vi "Actor Core.vi"(8 "error in":errorcluster, 11 "Launch IMAQ Display in":refnum<class "Launch File Viewer.lvclass">) -> (0 "error out":errorcluster={"status"=FALSE, "code"=0, "source"="Actor Framework.lvlib:Actor.lvclass:Launch Nested Actor.vi<APPEND>\n\n<b>Complete call chain:</b>\r\n     Actor Framework.lvlib:Actor.lvclass:Launch Nested Actor.vi\r\n     Launch HIJ FileViewer.lvlib:Launch File Viewer.lvclass:Actor Core.vi"}, 3 "Actor out":refnum<class "Actor.lvclass">)   [LabVIEW 2014, in "Launch HIJ FileViewer.lvlib" / "Launch File Viewer.lvclass"]
doc: "(<B>Filename</B>: Actor Framework.lvlib:Actor.lvclass:Actor Core.vi)\n\nReceives messages to the actor, reacts to them, and initiates any error handling that may shut the actor down.\n\nDescendant classes may override this VI to append parallel tasks for the actor to complete while it handles messages. Overrides use the Call Parent Method node."
uses:
  Launch File Viewer.lvclass
  <vilib>/ActorFramework/Actor/Actor.lvclass
  Analyze Actor/Analyze Actor/Analyze Actor.lvclass
  HIJ Vision Display/HIJ Vision Display Messages/New Results Msg/New Results Msg.lvclass
  HIJ Vision File Viewer/HIJ Vision File Viewer/HIJ Vision File Viewer.lvclass
  Results and Overlays/Results q-Factor/Analyze Results q-Factor.lvclass
  Analyze Classes/Analyze Fluence/Analyze Fluence.lvclass
  Results and Overlays/Results Fluence/Analyze Results Fluence.lvclass
  Results and Overlays/Results Base/Analyze Results Base.lvclass/Analyze Results Base.ctl
  HIJ Vision Display/HIJ Vision Display/HIJ Vision Display.lvclass/HIJ Vision Display.ctl
  Analyze Actor/Analyze Actor/Analyze Actor.lvclass/Analyze Actor.ctl
  <vilib>/ActorFramework/Actor/Actor.lvclass/Actor.ctl
  <vilib>/ActorFramework/Message Enqueuer/Message Enqueuer.lvclass/Message Enqueuer.ctl
  HIJ Vision Display/HIJ Vision Display Messages/Write Analyze Actor Msg/Write Analyze Enq Msg.lvclass/Write Analyze Enq Msg.ctl
  Shared Code/Viewable Actor/ViewableActor Messages/Insert Into SubPanel Msg/Insert Into SubPanel Msg.lvclass/Insert Into SubPanel Msg.ctl
  HIJ Vision File Viewer/HIJ Vision File Viewer Messages/Load Image from File Msg/Load Image from File Msg.lvclass/Load Image from File Msg.ctl
  Analyze Parameter/Analyze Parameter Energy/Analyze Parameter Energy.lvclass
  Analyze Parameter/Analyze Parameter Fluence/Analyze Parameter Fluence.lvclass
  Analyze Parameter/Analyze Parameter Energy/Analyze Parameter Energy.lvclass/Analyze Parameter Energy.ctl
  Analyze Actor/Analyze Actor Messages/Set Analyze Parameter Msg/Set Analyze Parameter Msg.lvclass/Set Analyze Parameter Msg.ctl
  Analyze Parameter/Analyze Parameter Energy/Write Energy.vi
  Results and Overlays/Results Base/Write Overlay_.vi
  Results and Overlays/Results Base/Write Overlay colors.vi
  HIJ Vision Display/HIJ Vision Display/Write Save Report_.vi
  HIJ Vision Display/HIJ Vision Display/Write Show ZoomBtn_.vi
  HIJ Vision Display/HIJ Vision Display/Write WorkDir.vi
  Analyze Actor/Analyze Actor/Write Analyze Objects.vi
  Analyze Actor/Analyze Actor/Write Publish Analyze Results Msg.vi
  Analyze Actor/Analyze Actor/Write Destination.vi
  <vilib>/ActorFramework/Message Enqueuer/Init from Existing Queue.vi
  <vilib>/ActorFramework/Message Enqueuer/Enqueue.vi
  <vilib>/ActorFramework/Message Priority Queue/Priority Enqueue.vi
  <vilib>/ActorFramework/Message Enqueuer/Message Enqueuer.lvclass
  HIJ Vision Display/HIJ Vision Display Messages/Write Analyze Actor Msg/Write Analyze Enq Msg.lvclass
  Shared Code/Viewable Actor/ViewableActor Messages/Insert Into SubPanel Msg/Insert Into SubPanel Msg.lvclass
  <vilib>/ActorFramework/Stop Msg/Stop Msg.lvclass
  HIJ Vision File Viewer/HIJ Vision File Viewer Messages/Load Image from File Msg/Load Image from File Msg.lvclass
  Analyze Actor/Analyze Actor Messages/Set Analyze Parameter Msg/Set Analyze Parameter Msg.lvclass
  HIJ Vision Display/HIJ Vision Display Messages/Evaluate with new Params Msg/Evaluate with new Params Msg.lvclass
  Shared Code/Viewable Actor/ViewableActor/ViewableActor.lvclass
panel:
  in  "Load Image Report":bool
  in  "Size of region (px)":i32=10
  in  "Energy":dbl[unit] format="%#_13g"
  in  "Image":path=path "C:/Users/user/Desktop/test/WorkDir"
  in  "Stop Button":bool=TRUE
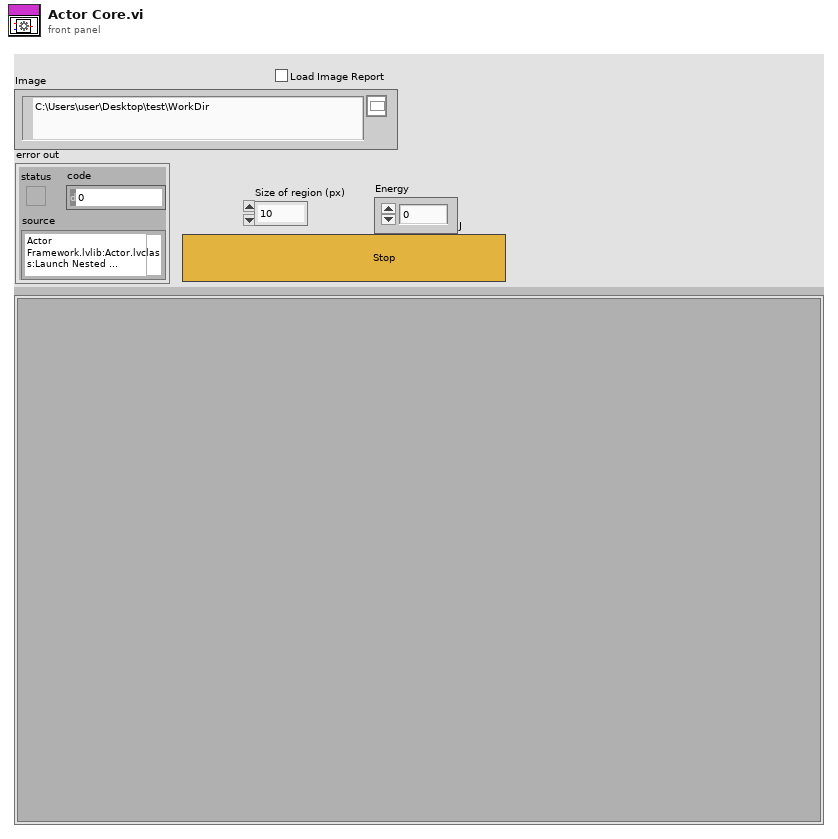
[diagram p1: front panel]
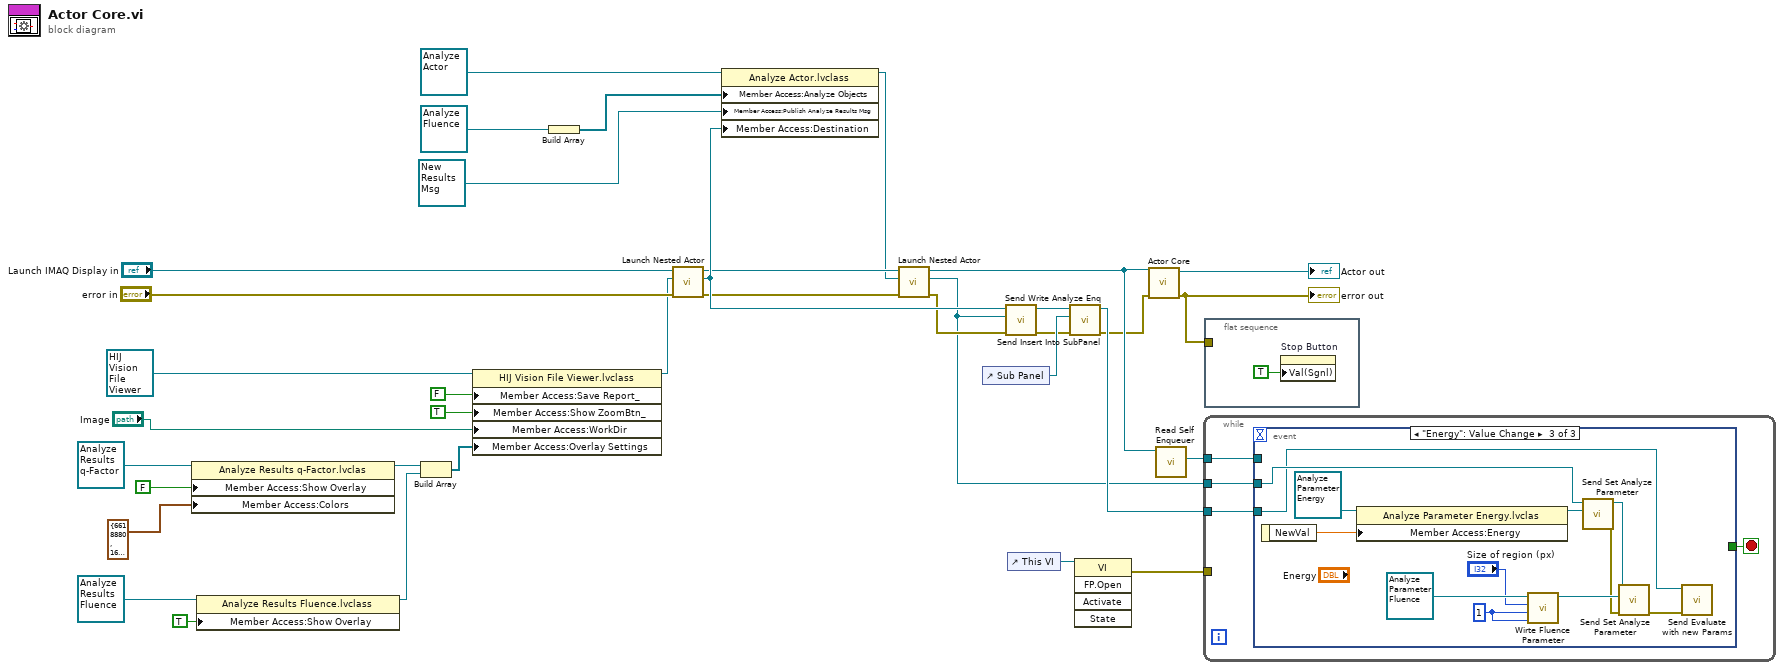
[diagram p0: block diagram]
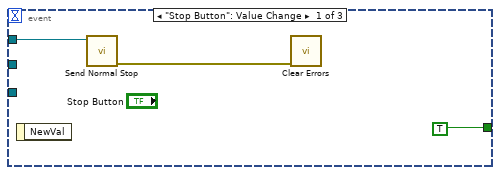
[diagram p2: hidden frame]
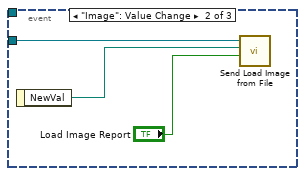
[diagram p3: hidden frame]
diagram:
  n1 = property class="Analyze Results q-Factor.lvclas"(reference=refnum<class "Analyze Results q-Factor.lvclass"> refnum ("Analyze Results q-Factor.lvclass"), "Member Access:Show Overlay"=FALSE ("bOverlay"), "Member Access:Colors"=cluster{"Border":u32, "Text":u32} {"Border"=6618880, "Text"=16448250} ("Colors")) -> (reference out=w9:refnum<class "Analyze Results q-Factor.lvclass">)  [unwired: 1 in, 1 out]
  n2 = property class="Analyze Results Fluence.lvclass"(reference=refnum<class "Analyze Results Fluence.lvclass"> refnum ("Analyze Results Fluence.lvclass"), "Member Access:Show Overlay"=TRUE ("Show Overlay")) -> (reference out=w1:refnum<class "Analyze Results Fluence.lvclass">)  [unwired: 1 in, 1 out]
  n3 = Build Array(w9, w1) -> (w11:refnum<class "Analyze Results Base.lvclass">[])
  n4 = property class="HIJ Vision File Viewer.lvclass"(reference=refnum<class "HIJ Vision File Viewer.lvclass"> refnum ("HIJ Vision File Viewer.lvlib:HIJ Vision File Viewer.lvclass"), "Member Access:Save Report_"=FALSE ("Save Report_"), "Member Access:Show ZoomBtn_"=TRUE ("Show ZoomBtn_"), "Member Access:WorkDir"="Image", "Member Access:Overlay Settings"=w11) -> (reference out=w24:refnum<class "HIJ Vision File Viewer.lvclass">)  [unwired: 1 in, 1 out]
  n5 = Build Array(refnum<class "Analyze Fluence.lvclass"> refnum ("Analyze.lvlib:Analyze Fluence.lvclass")) -> (w20:refnum<class "Analyze Fluence.lvclass">[])
  n6 = call <vilib>:"Launch Nested Actor.vi"("error in (no error)"="error in", "Nested Actor"=w24, "Caller Actor in"="Launch IMAQ Display in") -> ("error out"=w25:errorcluster, "Nested Actor's Enqueuer"=w36:refnum<class "Message Enqueuer.lvclass">, "Caller Actor out"=w18:refnum<class "Launch File Viewer.lvclass">)  [unwired: 6 in]
  n7 = property class="Analyze Actor.lvclass"(reference=refnum<class "Analyze Actor.lvclass"> refnum ("Analyze Actor.lvlib:Analyze Actor.lvclass"), "Member Access:Analyze Objects"=w20, "Member Access:Publish Analyze Results Msg"=refnum<class "New Results Msg.lvclass"> refnum ("HIJ Vision Display.lvlib:New Results Msg.lvclass"), "Member Access:Destination"=w36) -> (reference out=w16:refnum<class "Analyze Actor.lvclass">)  [unwired: 1 in, 1 out]
  n8 = call <vilib>:"Launch Nested Actor.vi"("error in (no error)"=w25, "Nested Actor"=w16, "Caller Actor in"=w18) -> ("error out"=w14:errorcluster, "Nested Actor's Enqueuer"=w5:refnum<class "Message Enqueuer.lvclass">, "Caller Actor out"=w17:refnum<class "Launch File Viewer.lvclass">)  [unwired: 6 in]
  n9 = control-ref of="Sub Panel"() -> (w34:refnum<vi>)
  n10 = call "Send Write Analyze Enq.vi"("error in (no error)"=w14, "Actor Framework:Message Enqueuer"=w5, "Message Enqueuer"=w36) -> ("error out"=w13:errorcluster, "Message Enqueuer out"=w15:refnum<class "Message Enqueuer.lvclass">)  [unwired: 7 in]
  n11 = control-ref of="This VI"() -> (w28:refnum<vi>)
  n12 = call "Send Insert Into SubPanel.vi"("error in (no error)"=w13, "SubPanel Ref"=w34, "Message Enqueuer"=w15) -> ("error out"=w12:errorcluster, "Message Enqueuer out"=w23:refnum<class "Message Enqueuer.lvclass">)  [unwired: 7 in]
  n13 = invoke class="VI" method="FP.Open"(reference=w28) -> (error out=w22:errorcluster)  [unwired: 4 in, 4 out]
  n14 = call-parent "Actor Core.vi"("error in"=w12, "Actor in"=w17) -> ("error out"=w33:errorcluster, "Actor out"=→"Actor out":refnum<class "Actor.lvclass">)  [unwired: 8 in]
  "error out" <- w33
  n15 = call <vilib>:"Read Self Enqueuer.vi"("Actor"=w17) -> ("Self Enqueuer"=w32:refnum<class "Message Enqueuer.lvclass">)  [unwired: 10 in]
  n16 = while {
    tunnel: w32 -> [w39]
    tunnel: w23 -> [w38]
    tunnel: w22 -> [_]
    tunnel: w5 -> [w37]
    stop <- w40 stop-if-true
    n17 = event shown="[2] \"Energy\": Value Change" {
      selector: _ -> [_ _ _]
      dyn-events: _ -> [_ _ _]
      timeout: _ -> [_ _ _]
      tunnel: [TRUE _ _] -> w40
      tunnel: w39 -> [w42 _ _]
      tunnel: w38 -> [_ w46 w55]
      tunnel: w37 -> [_ _ w56]
      event "Stop Button": Value Change {
        n18 = event-data() -> ()  [unwired: 1 in, 1 out]
        n19 = call <vilib>:"Send Normal Stop.vi"("Message Enqueuer"=w42) -> ("error out"=w41:errorcluster)  [unwired: 10 in]
        n20 = call <vilib>:"Clear Errors.vi"("error in (no error)"=w41) -> ()  [unwired: 5 in, 2 out]
      }
      event "Image": Value Change {
        n21 = event-data() -> ("NewVal"=w45:path)  [unwired: 1 in]
        n22 = call "Send Load Image from File.vi"("Load Report"="Load Image Report", "Path"=w45, "Message Enqueuer"=w46) -> ()  [unwired: 7 in, 2 out]
      }
      event "Energy": Value Change {
        w47 = 1 ("#of Areas")
        n23 = event-data() -> ("NewVal"=w58:dbl[unit])  [unwired: 1 in]
        n24 = property class="Analyze Parameter Energy.lvclas"(reference=refnum<class "Analyze Parameter Energy.lvclass"> refnum ("Analyze Parameter Energy.lvclass"), "Member Access:Energy"=w58) -> (reference out=w57:refnum<class "Analyze Parameter Energy.lvclass">)  [unwired: 1 in, 1 out]
        n25 = call "Wirte Fluence Parameter.vi"("#of Areas"=w47, "#Overlays"=w47, "Size of region (px)"="Size of region (px)", "Analyze Parameter Fluence in"=refnum<class "Analyze Parameter Fluence.lvclass"> refnum ("Analyze Parameter Fluence.lvclass")) -> ("Analyze Parameter Fluence out"=w52:refnum<class "Analyze Parameter Fluence.lvclass">)  [unwired: 7 in]
        n26 = call "Send Set Analyze Parameter.vi"("Analyze Parameter"=w57, "Message Enqueuer"=w56) -> ("error out"=w50:errorcluster, "Message Enqueuer out"=w51:refnum<class "Message Enqueuer.lvclass">)  [unwired: 8 in]
        n27 = call "Send Set Analyze Parameter.vi"("error in (no error)"=w50, "Analyze Parameter"=w52, "Message Enqueuer"=w51) -> ("error out"=w49:errorcluster)  [unwired: 7 in, 1 out]
        n28 = call "Send Evaluate with new Params.vi"("error in (no error)"=w49, "Message Enqueuer"=w55) -> ()  [unwired: 8 in, 2 out]
      }
    }
  }
  n29 = flat-sequence {
    tunnel: w33 -> [_]
    frame #0 {
      n30 = property on="Stop Button" class="Bool (strict)"("Val(Sgnl)"=TRUE) -> ()  [unwired: 2 in, 2 out]
    }
  }
